vi "ep_Add New Manufacturers.vi"(10 "manufacturer":string, 11 "manufacturers input":string[](array[string])) -> (3 "manufacturer output":string[](array[string]))   [LabVIEW 2011, in "NI_EP_COMTRADE.lvlib"]
uses:
  <vilib>/addons/Electrical Power/File IO/NI_EP_COMTRADE.lvlib
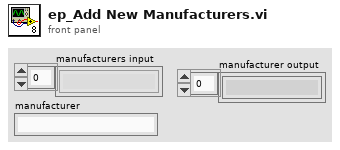
[diagram p1: front panel]
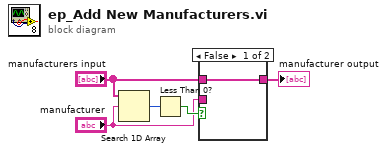
[diagram p0: block diagram]
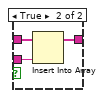
[diagram p2: hidden frame]
diagram:
  n1 = Search 1D Array(1D array="manufacturers input", element="manufacturer") -> (index of element=w5:i32)  [unwired: 1 in]
  n2 = Less Than 0?(x=w5) -> (x < 0?=w4:bool)
  n3 = case shown="False" w4 {
    tunnel: "manufacturers input" -> [w6 w9]
    tunnel: "manufacturer" -> [_ w8]
    tunnel: [w6 w7] -> w1
    frame False {
    }
    frame True {
      n4 = Insert Into Array(array=w9, new element=w8) -> (w7:string[])  [unwired: 1 in]
    }
  }
  "manufacturer output" <- w1
